vi "DataToFile.vi"(8 "error in (no error)":errorcluster, 10 "Sensor Index/\nSegment No.":u32, 11 "File Refnum in":refnum<file>) -> (0 "error out":errorcluster, 3 "File Refnum out":refnum<file>)   [LabVIEW 2018]
uses:
  globals/QC_RunInformation.vi
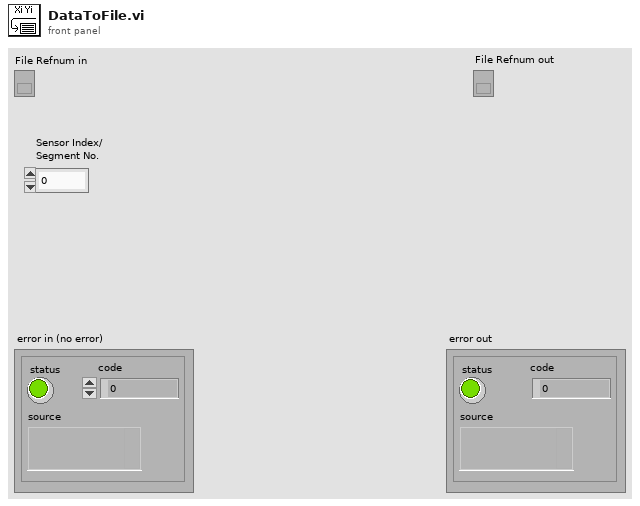
[diagram p1: front panel]
types:
  T1 = enum16{"Reset", "Read Array", "Read Element", "Write Element", "Write Array", "Add Element", "Add Array"}
  T2 = cluster{"Sensor Serial No.:":string, "Wafer:":string, "Batch:":string, "Manufacturer:":string, "Device Category:":string, "Database Serial No.:":string, "Date Initiated:":string, "Time Initiated:":string, "Test":string, "Probeplan used:":string, "End of Run comment:":string, "User:":string, "Vbias SMU":string, "LCR":string, "Test SMU":string, "Test DMM":string, "Comments":string, "Measurement results":cluster{"IV":string, "CV":string, "Cis":string, "Ris":string, "Stability":string, "PTP":string, "Striptest":string}}
  T3 = cluster{"Institute":string, "Manufacturers":string[], "Devices":string[], "Serialnumbers Lookup DB":string, "Data directory":string, "Backup & screenshot directory":string, "List of known users":string[], "Measurement switch not used":bool, "Measurement Switch":string, "DUT Switch":string, "Rseries IV [MOhm]":string, "Rshunt IV [MOhm]":string, "Rseries CV [MOhm]":string, "DC blocking Cap [µF]":string, "Rseries LCR [MOhm]":string, "Rseries stability [MOhm]":string, "Rshunt stability [MOhm]":string, "Rseries striptest bias [MOhm]":string, "Rseries strip pinhole [MOhm]":string}
  T4 = cluster{"Current Data":u32, "Data OUT":dbl, "Data OUT":dbl, dbl, "Data OUT":dbl}[]
  T5 = cluster{"Data OUT":dbl, "Data OUT":dbl, "Data OUT":dbl, dbl}[]
  T6 = cluster{"Data OUT":dbl, "Data OUT":dbl, "Data OUT":dbl}[]
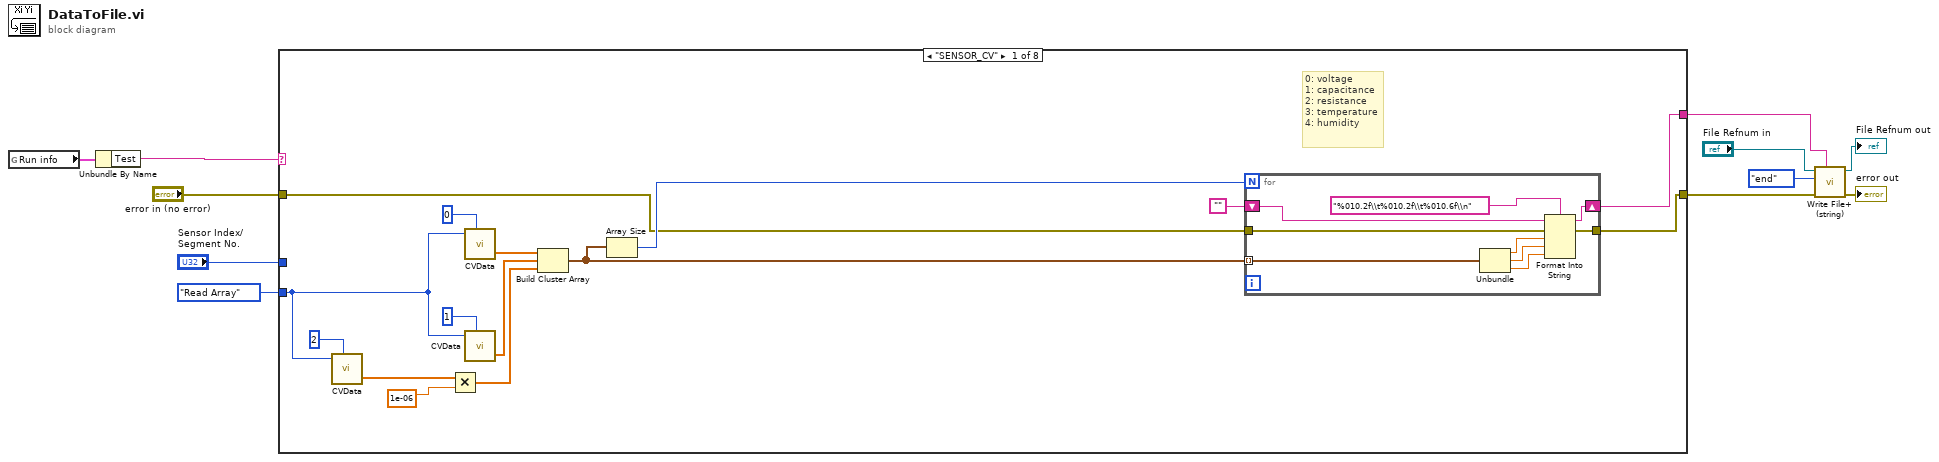
[diagram p0: block diagram]
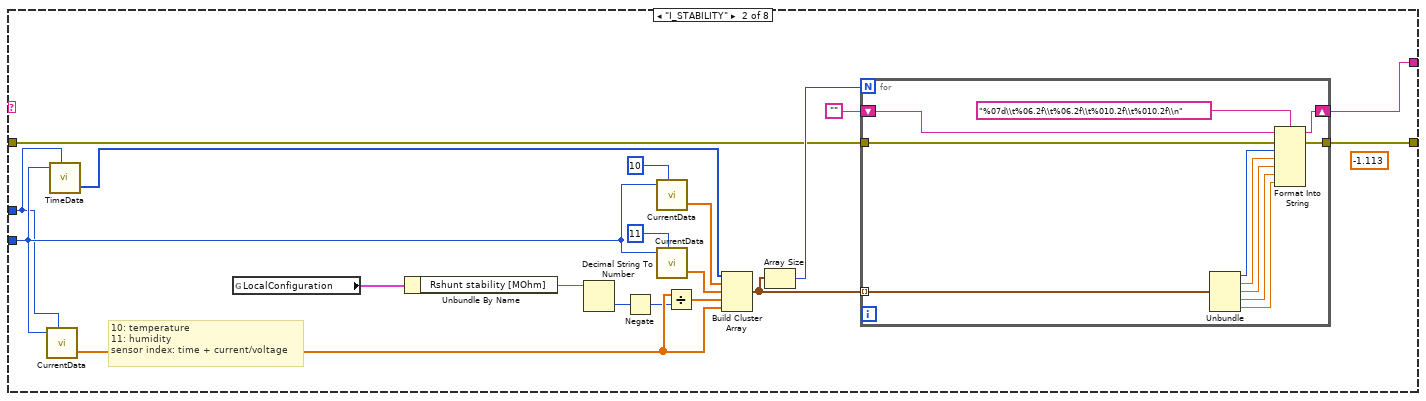
[diagram p2: hidden frame]
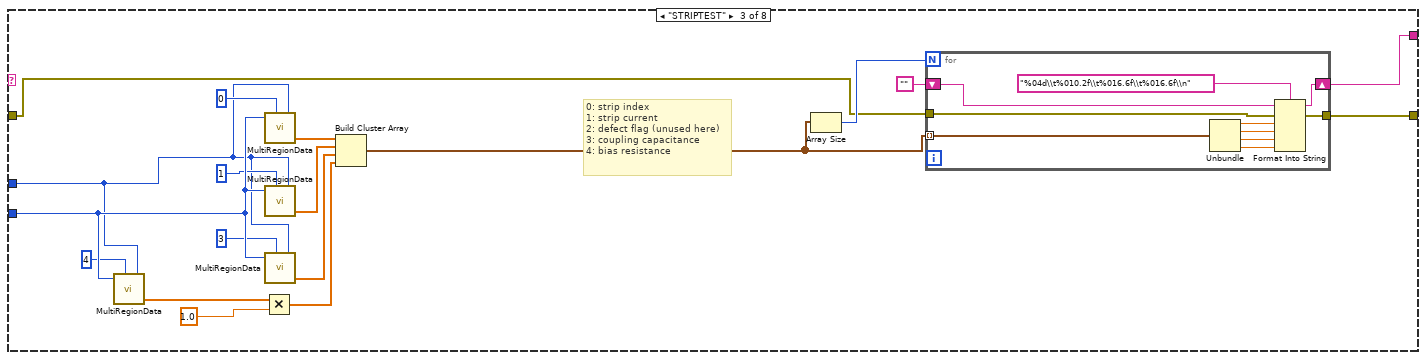
[diagram p3: hidden frame]
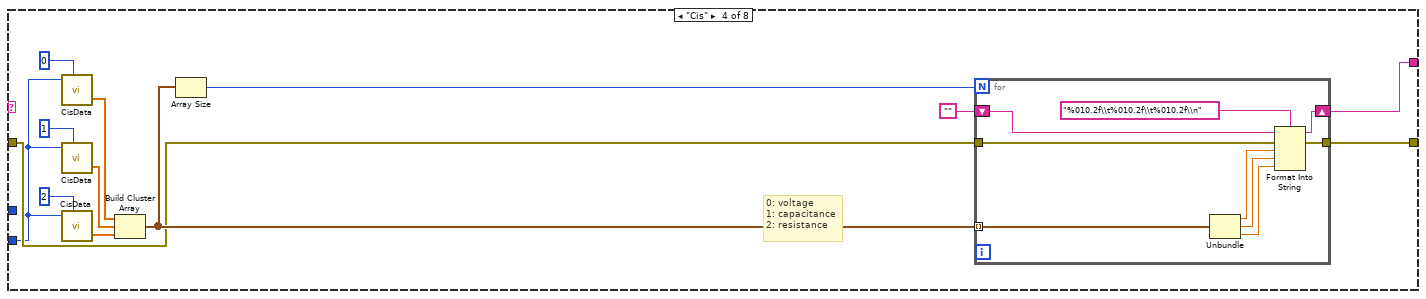
[diagram p4: hidden frame]
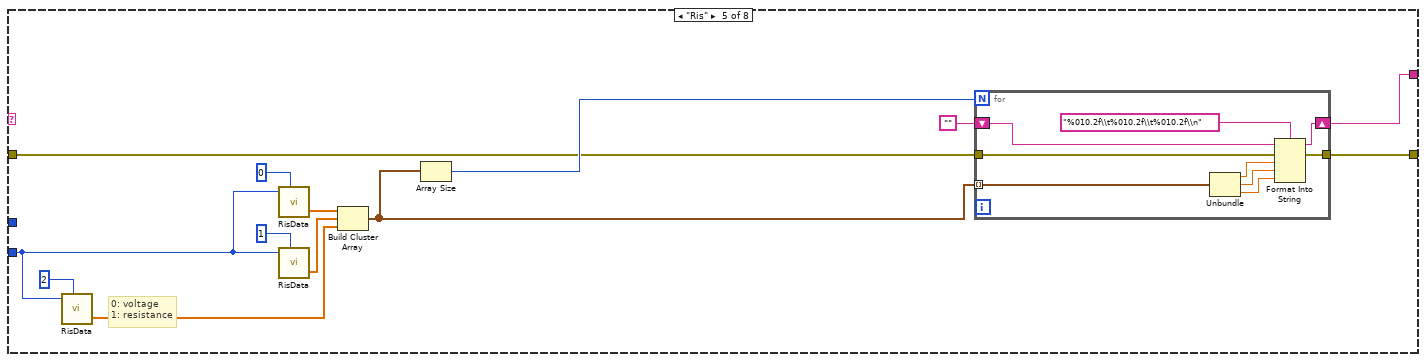
[diagram p5: hidden frame]
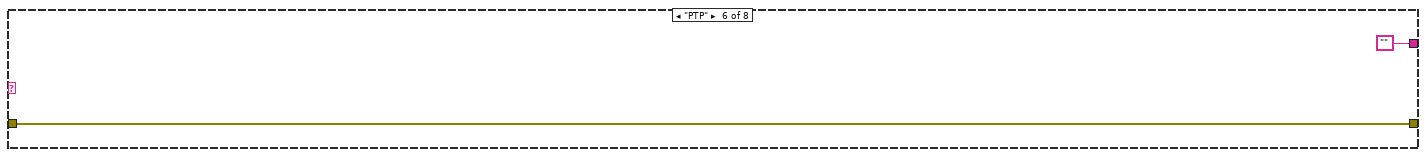
[diagram p6: hidden frame]
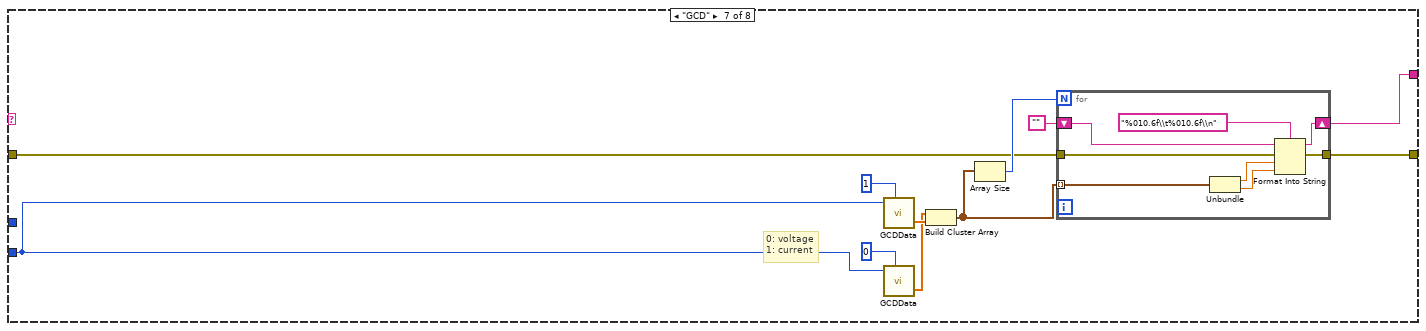
[diagram p7: hidden frame]
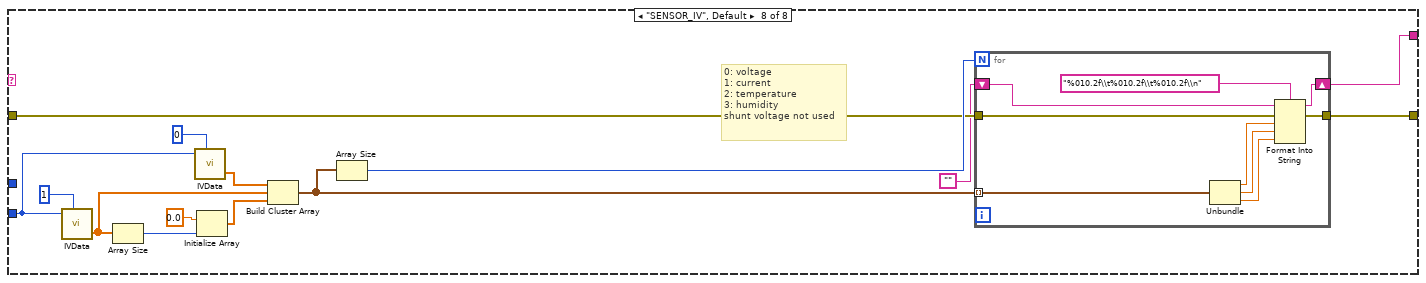
[diagram p8: hidden frame]
diagram:
  n1 = global read "QC_RunInformation.vi" "Run info"() -> (w11:T2)
  n2 = Unbundle By Name(w11) -> ("Test"=w10:string)
  n3 = case shown="\"SENSOR_CV\"" w10 {
    tunnel: T1."Read Array" ("Action") -> [w22 w52 w83 w97 w125 _ w146 w163]
    tunnel: [w16 w44 w68 w96 w117 "" w140 w167] -> w5
    tunnel: "error in (no error)" -> [w24 w46 w70 w104 w119 w138 w143 w166]
    tunnel: [w17 w45 w69 w95 w118 w138 w142 w165] -> w3
    tunnel: "Sensor Index/\nSegment No." -> [_ w43 w67 _ _ _ _ _]
    frame "SENSOR_CV" {
      # "0: voltage\n1: capacitance\n2: resistance\n3: temperature\n4: humidity"
      n4 = call "CVData.vi"("Action"=w22, "Array No."=u32 2 ("Action")) -> ("Array OUT"=w15:dbl[])  [unwired: 3 in, 1 out]
      n5 = Multiply(x=w15, y=1e-06) -> (x*y=w14:dbl[])
      n6 = call "CVData.vi"("Action"=w22, "Array No."=u32 0 ("Action")) -> ("Array OUT"=w18:dbl[])  [unwired: 3 in, 1 out]
      n7 = call "CVData.vi"("Action"=w22, "Array No."=u32 1 ("Action")) -> ("Array OUT"=w19:dbl[])  [unwired: 3 in, 1 out]
      n8 = Build Cluster Array(w18, w19, w14) -> (w26:cluster{"Data OUT":dbl, "Data OUT":dbl, dbl}[])
      n9 = Array Size(array=w26) -> (size(s)=w25:i32)
      n10 = for {
        N: w25 -> [_]
        tunnel: w26 -> [w35] mode=indexing
        tunnel: w24 -> [w30]
        tunnel: [w29] -> w17
        shift-right: [w31] -> w16
        shift-left: "" -> [w28]
        n11 = Unbundle(w35) -> ("Data OUT"=w34:dbl, "Data OUT"=w33:dbl, w27:dbl)
        n12 = Format Into String(format string="%010.2f\\t%010.2f\\t%010.6f\\n", initial string=w28, error in=w30, w34, w33, w27) -> (resulting string=w31:string, error out=w29:errorcluster)
      }
    }
    frame "I_STABILITY" {
      (unwired) -1.113
      # "10: temperature\n11: humidity\nsensor index: time + current/voltage"
      n13 = call "CurrentData.vi"("Action"=w52, "Array No."=w43) -> ("Array OUT"=w41:dbl[])  [unwired: 3 in, 1 out]
      n14 = call "TimeData.vi"("Action"=w52, "Array No."=w43) -> ("Array OUT"=w49:u32[])  [unwired: 3 in, 1 out]
      n15 = global read "QC_RunInformation.vi" "LocalConfiguration"() -> (w39:T3)
      n16 = Unbundle By Name(w39) -> ("Rshunt stability [MOhm]"=w38:string)
      n17 = Decimal String To Number(string=w38) -> (number=w37:i32)  [unwired: 2 in, 1 out]
      n18 = Negate(x=w37) -> (-x=w36:i32)
      n19 = call "CurrentData.vi"("Action"=w52, "Array No."=u32 10 ("Action")) -> ("Array OUT"=w48:dbl[])  [unwired: 3 in, 1 out]
      n20 = call "CurrentData.vi"("Action"=w52, "Array No."=u32 11 ("Action")) -> ("Array OUT"=w47:dbl[])  [unwired: 3 in, 1 out]
      n21 = Divide(x=w41, y=w36) -> (x/y=w40:dbl[])
      n22 = Build Cluster Array(w49, w48, w47, w40, w41) -> (w54:T4)
      n23 = Array Size(array=w54) -> (size(s)=w53:i32)
      n24 = for {
        N: w53 -> [_]
        tunnel: w54 -> [w65] mode=indexing
        tunnel: w46 -> [w60]
        tunnel: [w59] -> w45
        shift-right: [w61] -> w44
        shift-left: "" -> [w58]
        n25 = Unbundle(w65) -> ("Current Data"=w64:u32, "Data OUT"=w63:dbl, "Data OUT"=w57:dbl, w56:dbl, "Data OUT"=w55:dbl)
        n26 = Format Into String(format string="%07d\\t%06.2f\\t%06.2f\\t%010.2f\\t%010.2f\\n", initial string=w58, error in=w60, w64, w63, w57, w56, w55) -> (resulting string=w61:string, error out=w59:errorcluster)
      }
    }
    frame "STRIPTEST" {
      # "0: strip index\n1: strip current\n2: defect flag (unused here)\n3: coupling capacitance\n4: bias resistance"
      n27 = call "MultiRegionData.vi"("Action"=w83, "Array No."=u32 4 ("Action"), "Region index"=w67) -> ("Array OUT"=w77:dbl[])  [unwired: 3 in, 1 out]
      n28 = Multiply(x=w77, y=1.0) -> (x*y=w71:dbl[])
      n29 = call "MultiRegionData.vi"("Action"=w83, "Array No."=u32 0 ("Action"), "Region index"=w67) -> ("Array OUT"=w74:dbl[])  [unwired: 3 in, 1 out]
      n30 = call "MultiRegionData.vi"("Action"=w83, "Array No."=u32 1 ("Action"), "Region index"=w67) -> ("Array OUT"=w73:dbl[])  [unwired: 3 in, 1 out]
      n31 = call "MultiRegionData.vi"("Action"=w83, "Array No."=u32 3 ("Action"), "Region index"=w67) -> ("Array OUT"=w72:dbl[])  [unwired: 3 in, 1 out]
      n32 = Build Cluster Array(w74, w73, w72, w71) -> (w76:T5)
      n33 = Array Size(array=w76) -> (size(s)=w75:i32)
      n34 = for {
        N: w75 -> [_]
        tunnel: w76 -> [w93] mode=indexing
        tunnel: w70 -> [w88]
        tunnel: [w87] -> w69
        shift-right: [w89] -> w68
        shift-left: "" -> [w86]
        n35 = Unbundle(w93) -> ("Data OUT"=w92:dbl, "Data OUT"=w91:dbl, "Data OUT"=w85:dbl, w84:dbl)
        n36 = Format Into String(format string="%04d\\t%010.2f\\t%016.6f\\t%016.6f\\n", initial string=w86, error in=w88, w92, w91, w85, w84) -> (resulting string=w89:string, error out=w87:errorcluster)
      }
    }
    frame "Cis" {
      # "0: voltage\n1: capacitance\n2: resistance"
      n37 = call "CisData.vi"("Action"=w97, "Array No."=u32 0 ("Action")) -> ("Array OUT"=w103:dbl[])  [unwired: 3 in, 1 out]
      n38 = call "CisData.vi"("Action"=w97, "Array No."=u32 1 ("Action")) -> ("Array OUT"=w102:dbl[])  [unwired: 3 in, 1 out]
      n39 = call "CisData.vi"("Action"=w97, "Array No."=u32 2 ("Action")) -> ("Array OUT"=w101:dbl[])  [unwired: 3 in, 1 out]
      n40 = Build Cluster Array(w103, w102, w101) -> (w106:T6)
      n41 = Array Size(array=w106) -> (size(s)=w105:i32)
      n42 = for {
        N: w105 -> [_]
        tunnel: w106 -> [w115] mode=indexing
        tunnel: w104 -> [w110]
        tunnel: [w109] -> w95
        shift-right: [w111] -> w96
        shift-left: "" -> [w108]
        n43 = Unbundle(w115) -> ("Data OUT"=w114:dbl, "Data OUT"=w113:dbl, "Data OUT"=w107:dbl)
        n44 = Format Into String(format string="%010.2f\\t%010.2f\\t%010.2f\\n", initial string=w108, error in=w110, w114, w113, w107) -> (resulting string=w111:string, error out=w109:errorcluster)
      }
    }
    frame "Ris" {
      # "0: voltage\n1: resistance"
      n45 = call "RisData.vi"("Action"=w125, "Array No."=u32 2 ("Action")) -> ("Array OUT"=w120:dbl[])  [unwired: 3 in, 1 out]
      n46 = call "RisData.vi"("Action"=w125, "Array No."=u32 0 ("Action")) -> ("Array OUT"=w122:dbl[])  [unwired: 3 in, 1 out]
      n47 = call "RisData.vi"("Action"=w125, "Array No."=u32 1 ("Action")) -> ("Array OUT"=w121:dbl[])  [unwired: 3 in, 1 out]
      n48 = Build Cluster Array(w122, w121, w120) -> (w124:T6)
      n49 = Array Size(array=w124) -> (size(s)=w123:i32)
      n50 = for {
        N: w123 -> [_]
        tunnel: w124 -> [w137] mode=indexing
        tunnel: w119 -> [w132]
        tunnel: [w131] -> w118
        shift-right: [w133] -> w117
        shift-left: "" -> [w130]
        n51 = Unbundle(w137) -> ("Data OUT"=w136:dbl, "Data OUT"=w135:dbl, "Data OUT"=w129:dbl)
        n52 = Format Into String(format string="%010.2f\\t%010.2f\\t%010.2f\\n", initial string=w130, error in=w132, w136, w135, w129) -> (resulting string=w133:string, error out=w131:errorcluster)
      }
    }
    frame "PTP" {
    }
    frame "GCD" {
      # "0: voltage\n1: current"
      n53 = call "GCDData.vi"("Action"=w146, "Array No."=u32 1 ("Action")) -> ("Array OUT"=w145:dbl[])  [unwired: 3 in, 1 out]
      n54 = call "GCDData.vi"("Action"=w146, "Array No."=u32 0 ("Action")) -> ("Array OUT"=w144:dbl[])  [unwired: 3 in, 1 out]
      n55 = Build Cluster Array(w144, w145) -> (w150:cluster{"Data OUT":dbl, "Data OUT":dbl}[])
      n56 = Array Size(array=w150) -> (size(s)=w149:i32)
      n57 = for {
        N: w149 -> [_]
        tunnel: w150 -> [w158] mode=indexing
        tunnel: w143 -> [w153]
        tunnel: [w152] -> w142
        shift-right: [w154] -> w140
        shift-left: "" -> [w151]
        n58 = Unbundle(w158) -> ("Data OUT"=w157:dbl, "Data OUT"=w156:dbl)
        n59 = Format Into String(format string="%010.6f\\t%010.6f\\n", initial string=w151, error in=w153, w157, w156) -> (resulting string=w154:string, error out=w152:errorcluster)
      }
    }
    frame "SENSOR_IV", Default {
      # "0: voltage\n1: current\n2: temperature\n3: humidity\nshunt voltage not used"
      n60 = call "IVData.vi"("Action"=w163, "Array No."=u32 1 ("Action")) -> ("Array OUT"=w162:dbl[])  [unwired: 3 in, 1 out]
      n61 = Array Size(array=w162) -> (size(s)=w160:i32)
      n62 = call "IVData.vi"("Action"=w163, "Array No."=u32 0 ("Action")) -> ("Array OUT"=w170:dbl[])  [unwired: 3 in, 1 out]
      n63 = Initialize Array(0.0, w160) -> (w159:dbl[])
      n64 = Build Cluster Array(w170, w162, w159) -> (w169:cluster{"Data OUT":dbl, "Data OUT":dbl, dbl}[])
      n65 = Array Size(array=w169) -> (size(s)=w168:i32)
      n66 = for {
        N: w168 -> [_]
        tunnel: w169 -> [w181] mode=indexing
        tunnel: w166 -> [w176]
        tunnel: [w175] -> w165
        shift-right: [w177] -> w167
        shift-left: "" -> [w174]
        n67 = Unbundle(w181) -> ("Data OUT"=w180:dbl, "Data OUT"=w179:dbl, w173:dbl)
        n68 = Format Into String(format string="%010.2f\\t%010.2f\\t%010.2f\\n", initial string=w174, error in=w176, w180, w179, w173) -> (resulting string=w177:string, error out=w175:errorcluster)
      }
    }
  }
  n69 = call <vilib>:"Write File+ (string).vi"("string"=w5, "error in (no error)"=w3, "pos mode (rel. to end:1)"=enum16{"start", "end", "current"}."end", "refnum"="File Refnum in") -> ("error out"=→"error out":errorcluster, "dup refnum"=→"File Refnum out":refnum<file>)  [unwired: 3 in, 1 out]
